vi "Day 02 (Part One).vi"() -> ()   [LabVIEW 2021]
panel:
  out "result":i32
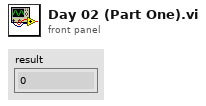
[diagram p1: front panel]
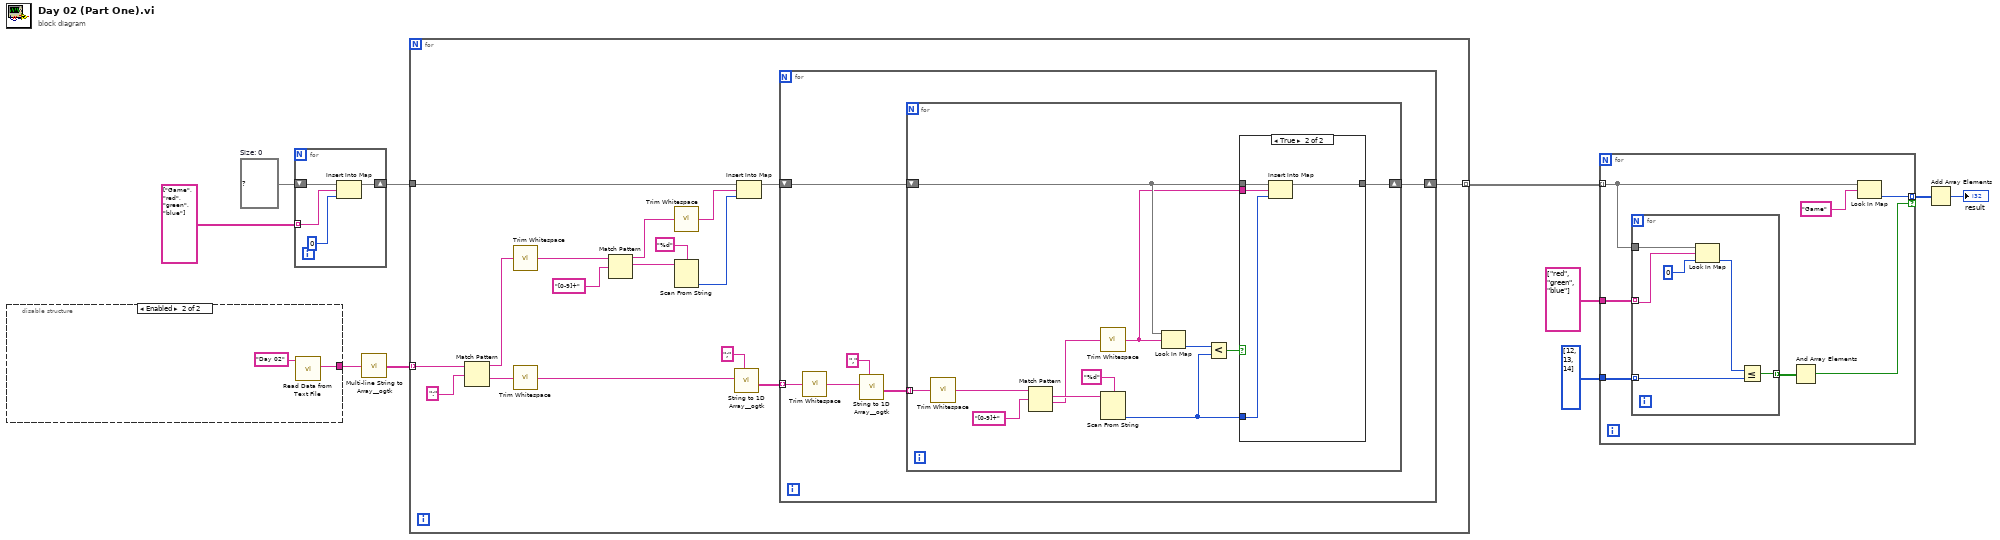
[diagram p0: block diagram]
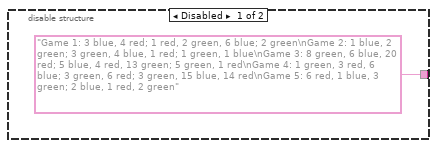
[diagram p3: hidden frame]
diagram:
  w7 = map{string, i32} {}  # Size: 0
  n1 = disable-structure shown="Enabled" {
    disable-tunnel: ["Game 1: 3 blue, 4 red; 1 red, 2 green, 6 blue; 2 green\nGame 2: 1 blue, 2 green; 3 green, 4 blue, 1 red; 1 green, 1 blue\nGame 3: 8 green, 6 blue, 20 red; 5 blue, 4 red, 13 green; 5 green, 1 red\nGame 4: 1 green, 3 red, 6 blue; 3 green, 6 red; 3 green, 15 blue, 14 red\nGame 5: 6 red, 1 blue, 3 green; 2 blue, 1 red, 2 green" w13] -> w10
    frame Disabled {
    }
    frame Enabled {
      n2 = call "Read Data from Text File.vi"("Subfolder"="Day 02") -> ("data"=w13:string)  [unwired: 10 in]
    }
  }
  n3 = for {
    tunnel: string[] ["Game", "red", "green", "blue"] -> [w17] mode=indexing
    shift-right: [w14] -> w6
    shift-left: w7 -> [w15]
    n4 = Insert Into Map(map in=w15, key=w17, value=0) -> (map out=w14:map{string, i32})  [unwired: 2 out]
  }
  n5 = call <userlib>:"Multi-line String to Array__ogtk.vi"("string"=w10) -> ("lines"=w9:string[])
  n6 = for {
    tunnel: w9 -> [w34] mode=indexing
    tunnel: w6 -> [w27]
    tunnel: [w18] -> w5 mode=indexing
    n7 = Match Pattern(string=w34, regular expression=":") -> (before substring=w32:string, after substring=w31:string)  [unwired: 1 in, 2 out]
    n8 = call <vilib>:"Trim Whitespace.vi"("string"=w32) -> ("trimmed string"=w25:string)  [unwired: 1 in]
    n9 = call <vilib>:"Trim Whitespace.vi"("string"=w31) -> ("trimmed string"=w30:string)  [unwired: 1 in]
    n10 = Match Pattern(string=w25, regular expression="[0-9]+") -> (before substring=w23:string, match substring=w22:string)  [unwired: 1 in, 2 out]
    n11 = call <vilib>:"Trim Whitespace.vi"("string"=w23) -> ("trimmed string"=w20:string)  [unwired: 1 in]
    n12 = Scan From String(format string="%d", input string=w22) -> (output 1=w21:i32)  [unwired: 3 in, 3 out]
    n13 = call <userlib>:"String to 1D Array__ogtk.vi"("delimiter (Tab)"=";", "string"=w30) -> ("Array of Strings"=w28:string[])  [unwired: 9 in]
    n14 = Insert Into Map(map in=w27, key=w20, value=w21) -> (map out=w19:map{string, i32})  [unwired: 2 out]
    n15 = for {
      tunnel: w28 -> [w40] mode=indexing
      shift-right: [w35] -> w18
      shift-left: w19 -> [w36]
      n16 = call <vilib>:"Trim Whitespace.vi"("string"=w40) -> ("trimmed string"=w38:string)  [unwired: 1 in]
      n17 = call <userlib>:"String to 1D Array__ogtk.vi"("delimiter (Tab)"=",", "string"=w38) -> ("Array of Strings"=w37:string[])  [unwired: 9 in]
      n18 = for {
        tunnel: w37 -> [w52] mode=indexing
        shift-right: [w41] -> w35
        shift-left: w36 -> [w44]
        n19 = call <vilib>:"Trim Whitespace.vi"("string"=w52) -> ("trimmed string"=w51:string)  [unwired: 1 in]
        n20 = Match Pattern(string=w51, regular expression="[0-9]+") -> (match substring=w49:string, after substring=w47:string)  [unwired: 1 in, 2 out]
        n21 = call <vilib>:"Trim Whitespace.vi"("string"=w47) -> ("trimmed string"=w43:string)  [unwired: 1 in]
        n22 = Scan From String(format string="%d", input string=w49) -> (output 1=w42:i32)  [unwired: 3 in, 3 out]
        n23 = Look In Map(map=w44, key=w43) -> (value=w46:i32)  [unwired: 1 in, 1 out]
        n24 = Less?(x=w46, y=w42) -> (x < y?=w45:bool)
        n25 = case shown="True" w45 {
          tunnel: w44 -> [w53 w57]
          tunnel: w43 -> [_ w56]
          tunnel: w42 -> [_ w55]
          tunnel: [w53 w54] -> w41
          frame False {
          }
          frame True {
            n26 = Insert Into Map(map in=w57, key=w56, value=w55) -> (map out=w54:map{string, i32})  [unwired: 2 out]
          }
        }
      }
    }
  }
  n27 = for {
    tunnel: w5 -> [w61] mode=indexing
    tunnel: string[] ["red", "green", "blue"] -> [w64]
    tunnel: i32[] [12, 13, 14] -> [w63]
    tunnel: [w59] -> w2 mode=indexing if=w58
    n28 = for {
      tunnel: w61 -> [w70]
      tunnel: w64 -> [w69] mode=indexing
      tunnel: w63 -> [w66] mode=indexing
      tunnel: [w65] -> w62 mode=indexing
      n29 = Look In Map(map=w70, key=w69, default value=0) -> (value=w67:i32)  [unwired: 1 out]
      n30 = Less Or Equal?(x=w67, y=w66) -> (x <= y?=w65:bool)
    }
    n31 = And Array Elements(Boolean array=w62) -> (logical AND=w58:bool)
    n32 = Look In Map(map=w61, key="Game") -> (value=w59:i32)  [unwired: 1 in, 1 out]
  }
  n33 = Add Array Elements(numeric array=w2) -> (sum=→"result":i32)
